vi "Controller Read Inputs.vi"(8 "error in (no error)":errorcluster, 9 "PS Status Variables":refnum<k21>[](array[refnum]), 10 "PS Reading Variables":refnum<k21>[](array[refnum]), 11 "BPM Variables":refnum<k21>[](array[refnum])) -> (0 "error out":errorcluster, 1 "PS Status (per PS Rack)":u8[](array[numeric]), 2 "PS Readings":dbl[](array[numeric]), 3 "BPM Readings":dbl[](array[numeric]))   [LabVIEW 2011, in "Controller VIs.lvlib"]
doc: "Read all input variables from the Acquisition and Actuation chassis."
uses:
  Controller VIs.lvlib
  Simulated Beam VIs/Simulated PS Current.vi
  Simulated Beam VIs.lvlib
  Simulated Beam VIs/Simulated Beam Response.vi
  <vilib>/Analysis/NI_AALBase.lvlib
  <vilib>/ptbypt/NI_PtbyPt.lvlib
  <vilib>/Analysis/baseanly.llb/A x Vector.vi
panel:
  in  "BPM noise std":dbl=0.005 step=0.001
  in  "PS noise std":dbl=0.001 step=0.001
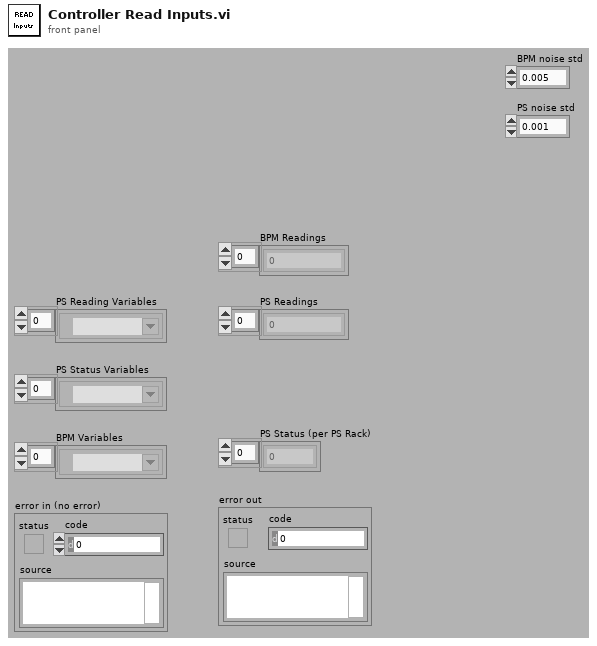
[diagram p1: front panel]
types:
  T1 = cluster{"filter structure":enum32{"IIR 2nd Order", "IIR 4th Order"}, "Reverse Coefficients":dbl[], "Forward Coefficients":dbl[]}
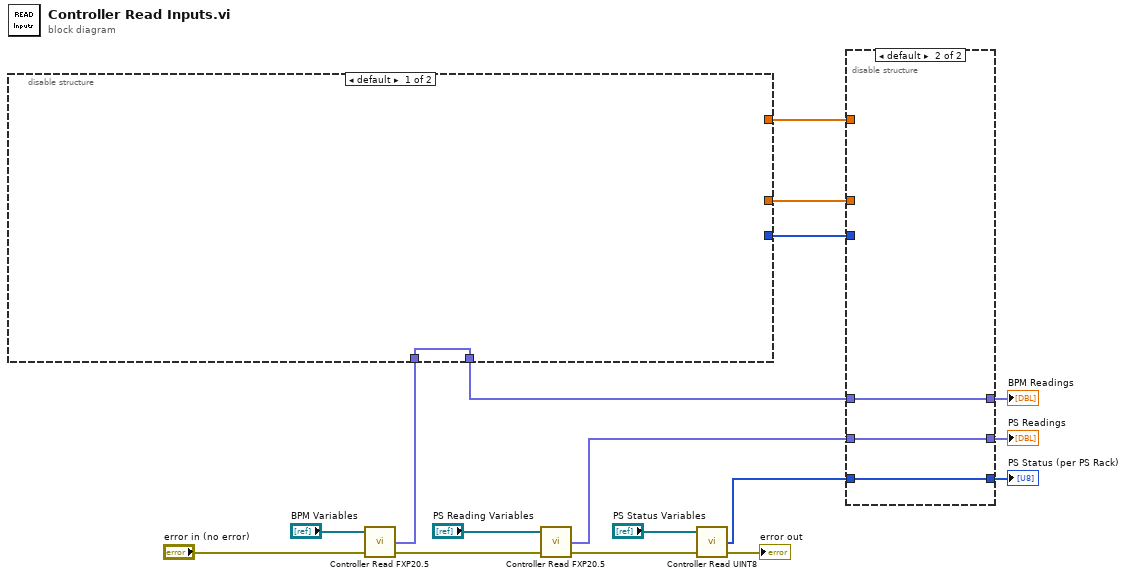
[diagram p0: block diagram]
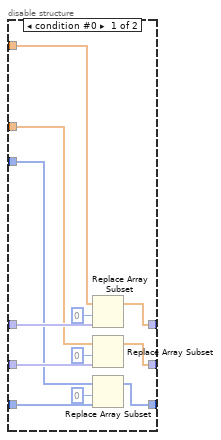
[diagram p2: hidden frame]
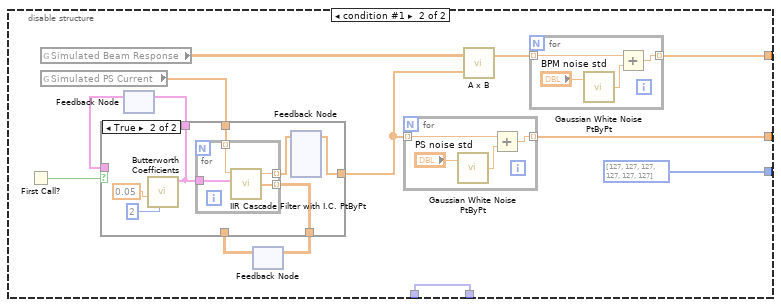
[diagram p3: hidden frame]
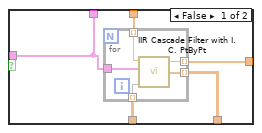
[diagram p4: hidden frame]
diagram:
  n1 = call "Controller Read FXP20.5.vi"("error in (no error)"="error in (no error)", "Variables"="BPM Variables") -> ("error out"=w12:errorcluster, "Values"=w5:fxp<+/-,20,5>[])  [unwired: 2 in]
  n2 = disable-structure shown="default" {
    disable-tunnel: [_ u8[] [127, 127, 127, 127, 127, 127] ("PS Status (per PS Rack)")] -> w1
    disable-tunnel: [_ w22] -> w2
    disable-tunnel: [_ w21] -> w3
    disable-tunnel: [w18 w20] -> w4
    disable-tunnel: w5 -> [w18 w20]
    frame condition #0 (active) {
    }
    frame condition #1 {
      n3 = First Call?() -> (First Call?: T/F=w30:bool)
      n4 = global read "Simulated Beam Response.vi" "Simulated Beam Response"() -> (w31:dbl[][])
      n5 = global read "Simulated PS Current.vi" "Simulated PS Current"() -> (w28:dbl[])
      n6 = feedback #1() -> (w27:T1)  [unwired: 1 in]
      n7 = feedback #2() -> (w24:dbl[][])  [unwired: 1 in]
      n8 = case shown="True" w30 {
        tunnel: w27 -> [w33 _]
        tunnel: w28 -> [w32 w46]
        tunnel: [w33 w45] -> w26
        tunnel: [w36 w43] -> w19
        tunnel: [w35 w44] -> w25
        tunnel: w24 -> [w34 _]
        frame False {
          n9 = for {
            tunnel: w33 -> [w41]
            tunnel: [w40] -> w35 mode=indexing
            tunnel: [w39] -> w36 mode=indexing
            tunnel: w34 -> [w38] mode=indexing
            tunnel: w32 -> [w37] mode=indexing
            n10 = call <vilib>:"IIR Cascade Filter with I.C. PtByPt.vi"("x"=w37, "IIR Filter Cluster"=w41, "Initial Condition"=w38) -> ("Filtered x"=w39:dbl, "Final Condition"=w40:dbl[])  [unwired: 2 in, 1 out]
          }
        }
        frame True {
          n11 = call <vilib>:"Butterworth Coefficients.vi"("order"=2, "low cutoff freq: fl"=0.05) -> ("IIR Filter Cluster"=w45:T1)  [unwired: 8 in, 1 out]
          n12 = for {
            tunnel: w45 -> [w52]
            tunnel: [w51] -> w44 mode=indexing
            tunnel: w46 -> [w50] mode=indexing
            tunnel: [w49] -> w42 mode=indexing
            n13 = call <vilib>:"IIR Cascade Filter with I.C. PtByPt.vi"("x"=w50, "IIR Filter Cluster"=w52) -> ("Filtered x"=w49:dbl, "Final Condition"=w51:dbl[])  [unwired: 3 in, 1 out]
          }
          n14 = feedback #3() -> (w43:dbl[])  [unwired: 1 in]
          n15 = feedback-in #3(w42) -> ()
        }
      }
      n16 = feedback-in #1(w26) -> ()
      n17 = feedback-in #2(w25) -> ()
      n18 = for {
        tunnel: [w55] -> w22 mode=indexing
        tunnel: w19 -> [w56] mode=indexing
        n19 = call <vilib>:"Gaussian White Noise PtByPt.vi"("standard deviation"="PS noise std") -> ("Gaussian white noise"=w53:dbl)  [unwired: 2 in]
        n20 = Add(x=w56, y=w53) -> (x+y=w55:dbl)
      }
      n21 = call-poly <vilib>:"A x B.vi"("Vector"=w19, "A"=w31) -> ("A x Vector"=w29:dbl[])  [unwired: 1 out]
      n22 = for {
        tunnel: [w59] -> w21 mode=indexing
        tunnel: w29 -> [w60] mode=indexing
        n23 = call <vilib>:"Gaussian White Noise PtByPt.vi"("standard deviation"="BPM noise std") -> ("Gaussian white noise"=w57:dbl)  [unwired: 2 in]
        n24 = Add(x=w60, y=w57) -> (x+y=w59:dbl)
      }
    }
  }
  n25 = call "Controller Read FXP20.5.vi"("error in (no error)"=w12, "Variables"="PS Reading Variables") -> ("error out"=w11:errorcluster, "Values"=w9:fxp<+/-,20,5>[])  [unwired: 2 in]
  n26 = call "Controller Read UINT8.vi"("error in (no error)"=w11, "Variables"="PS Status Variables") -> ("error out"=→"error out":errorcluster, "Values"=w6:u8[])  [unwired: 2 in]
  n27 = disable-structure shown="default" {
    disable-tunnel: [w69 w75] -> w10
    disable-tunnel: w4 -> [w71 w75]
    disable-tunnel: w9 -> [w65 w74]
    disable-tunnel: [w67 w74] -> w8
    disable-tunnel: [w61 w73] -> w7
    disable-tunnel: w6 -> [w62 w73]
    disable-tunnel: w3 -> [w72 _]
    disable-tunnel: w2 -> [w64 _]
    disable-tunnel: w1 -> [w63 _]
    frame condition #0 {
      n28 = Replace Array Subset(array=w72, new element=w71, index=0) -> (w69:dbl[])
      n29 = Replace Array Subset(array=w64, new element=w65, index=0) -> (w67:dbl[])
      n30 = Replace Array Subset(array=w63, new element=w62, index=0) -> (w61:u8[])
    }
    frame condition #1 (active) {
    }
  }
  "BPM Readings" <- w10
  "PS Readings" <- w8
  "PS Status (per PS Rack)" <- w7
